vi "Set ROI.vi"(8 "error in (no error)":errorcluster) -> (0 "error out":errorcluster)   [LabVIEW 2023, in "CameraOptionsInterface.lvclass"]
uses:
  CameraOptionsInterface.lvclass
panel:
  out "CameraOptionsInterface.lvclass":refnum<class "CameraOptionsInterface.lvclass">
  in  "CameraOptionsInterface.lvclass":refnum<class "CameraOptionsInterface.lvclass">
  in  "ROI":i32[](array[numeric])
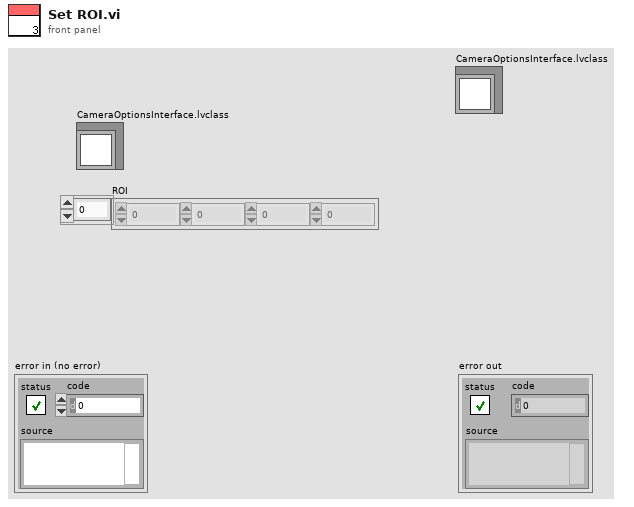
[diagram p1: front panel]
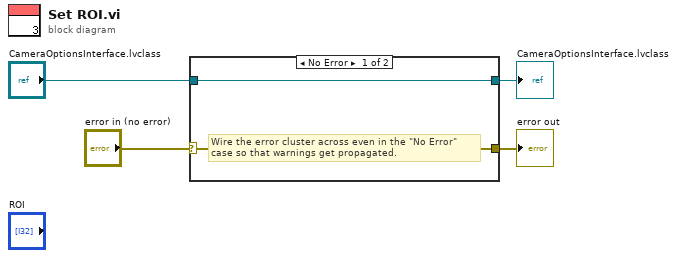
[diagram p0: block diagram]
diagram:
  n1 = case shown="No Error" "error in (no error)" {
    selector: "error in (no error)" -> [w5 w8]
    tunnel: [w5 w8] -> w3
    tunnel: [w6 w7] -> w2
    tunnel: "CameraOptionsInterface.lvclass" -> [w6 w7]
    frame No Error {
      # "Wire the error cluster across even in the \"No Error\"\ncase so that warnings get propagated."
    }
    frame Error {
    }
  }
  "error out" <- w3
  "CameraOptionsInterface.lvclass" <- w2
